vi "Off_Asc&DTCE.vi"(2 "Timeout (ms)":i32=40000000, 3 "connection ID in":refnum<k5>) -> (0 "Timeout (ms) 2":i32=40000000, 1 "connection ID out":refnum<k5>)   [LabVIEW 2016]
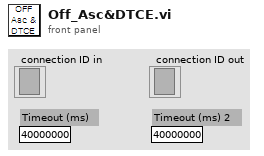
[diagram p1: front panel]
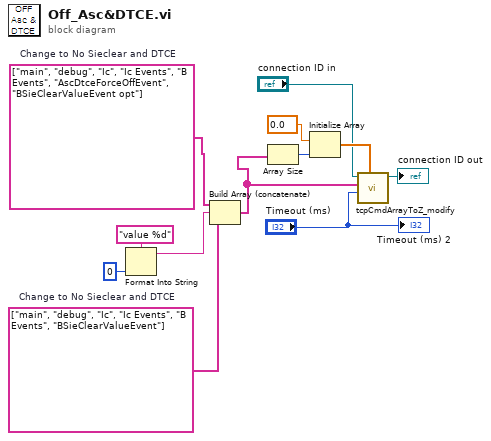
[diagram p0: block diagram]
diagram:
  w1 = string[] ["main", "debug", "Ic", "Ic Events", "B Events", "BSieClearValueEvent"]  # Change to No Sieclear and DTCE
  w5 = string[] ["main", "debug", "Ic", "Ic Events", "B Events", "AscDtceForceOffEvent", "BSieClearValueEvent opt"]  # Change to No Sieclear and DTCE
  n1 = Format Into String(format string="value %d", 0 ("입력 1")) -> (resulting string=w3:string)  [unwired: 2 in, 1 out]
  n2 = Build Array (concatenate)(w5, w3, w1) -> (w6:string[])
  n3 = Array Size(array=w6) -> (size(s)=w12:i32)
  n4 = Initialize Array(0.0 ("element"), w12) -> (w10:dbl[])
  n5 = call "tcpCmdArrayToZ_modify.vi"("Delay (sec)"=w10, "Timeout (ms)"="Timeout (ms)", "Command array"=w6, "connection ID in"="connection ID in") -> ("connection ID out"=→"connection ID out":refnum<k5>)  [unwired: 3 in, 4 out]
  "Timeout (ms) 2" <- "Timeout (ms)"
